vi "Array_size.vi"() -> ()   [LabVIEW 2024]
panel:
  out "size(s)":i32
  out "Array":dbl[](array[numeric])
  in  "Numeric":i32
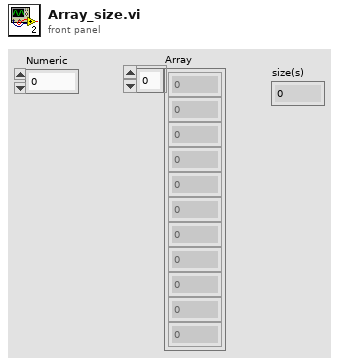
[diagram p1: front panel]
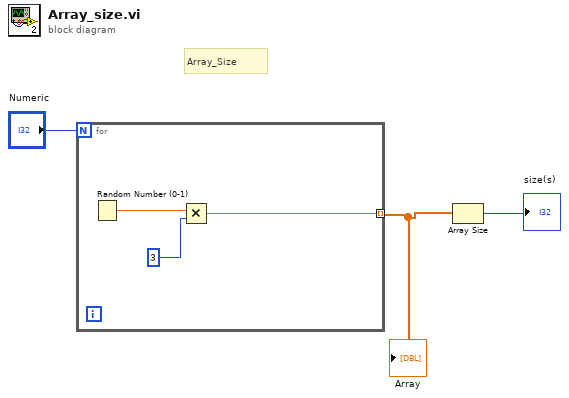
[diagram p0: block diagram]
diagram:
  # "Array_Size"
  n1 = for {
    N: "Numeric" -> [_]
    tunnel: [w4] -> w2 mode=indexing
    n2 = Random Number (0-1)() -> (number: 0 to 1=w6:dbl)
    n3 = Multiply(x=w6, y=3) -> (x*y=w4:dbl)
  }
  "Array" <- w2
  n4 = Array Size(array=w2) -> (size(s)=→"size(s)":i32)
